vi "rtin_ControlNslMux.vi"(7 "Set":bool, 8 "error in":errorcluster, 10 "axis in":u8, 11 "connection ID":refnum<k5>) -> (0 "error out":errorcluster, 2 "axis out":i32, 3 "connection ID":refnum<k5>)   [LabVIEW 2016, in "AMC_VIs.lvlib"]
uses:
  AMC_VIs.lvlib
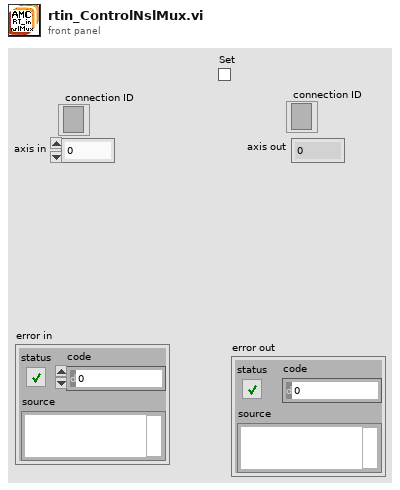
[diagram p1: front panel]
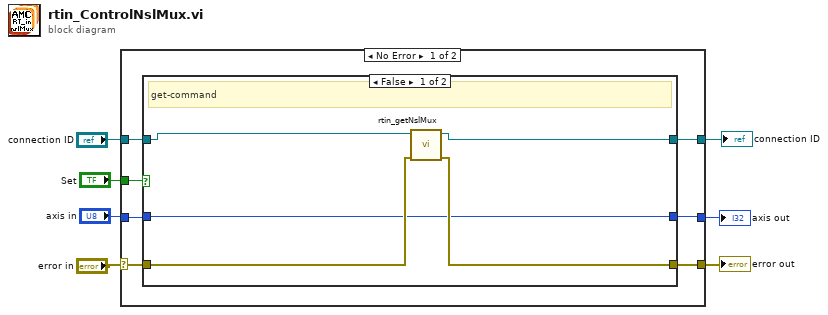
[diagram p0: block diagram]
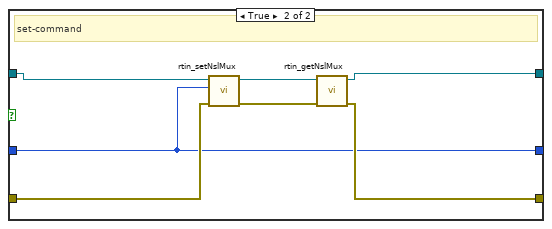
[diagram p2: hidden frame]
diagram:
  n1 = case shown="No Error" "error in" {
    selector: "error in" -> [w11 w29]
    tunnel: "axis in" -> [w14 w27]
    tunnel: [w10 w29] -> w6
    tunnel: "Set" -> [w12 _]
    tunnel: [w9 w28] -> w4
    tunnel: "connection ID" -> [w13 w28]
    tunnel: [w8 w27] -> w1
    frame No Error {
      n2 = case shown="False" w12 {
        tunnel: w13 -> [w19 w21]
        tunnel: w14 -> [w15 w20]
        tunnel: w11 -> [w16 w24]
        tunnel: [w17 w23] -> w10
        tunnel: [w18 w22] -> w9
        tunnel: [w15 w20] -> w8
        frame False {
          # "get-command"
          n3 = call "rtin_getNslMux.vi"("error in"=w16, "connection ID"=w19) -> ("error out"=w17:errorcluster, "connection ID"=w18:refnum<k5>)  [unwired: 8 in]
        }
        frame True {
          # "set-command"
          n4 = call "rtin_setNslMux.vi"("error in"=w24, "mux_mode"=w20, "connection ID"=w21) -> ("error out"=w26:errorcluster, "connection ID"=w25:refnum<k5>)  [unwired: 7 in]
          n5 = call "rtin_getNslMux.vi"("error in"=w26, "connection ID"=w25) -> ("error out"=w23:errorcluster, "connection ID"=w22:refnum<k5>)  [unwired: 8 in]
        }
      }
    }
    frame Error {
    }
  }
  "error out" <- w6
  "axis out" <- w1
  "connection ID" <- w4
